vi "Report to logger.vi"(8 "error in (no error)":errorcluster, 10 "Comment":string, 11 "Camera Actor in":refnum<class "Camera Actor.lvclass">) -> (0 "error out":errorcluster, 3 "Camera Actor out":refnum<class "Camera Actor.lvclass">)   [LabVIEW 2020, in "Camera Actor.lvlib" / "Camera Actor.lvclass"]
uses:
  Camera Actor.lvclass
  Camera Actor.lvclass/Camera Actor.ctl
  Logbook/Logbook/Logbook.lvclass
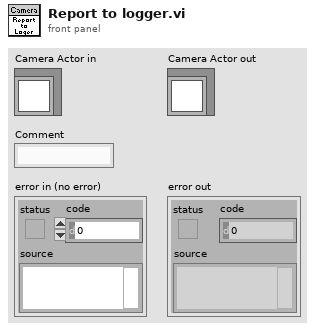
[diagram p1: front panel]
types:
  T1 = typedef "Camera Actor.lvlib/Camera Actor.lvclass/Operation Mode.ctl" = enum16{"Run", "Stop", "Exit", "Error", "Restart"}
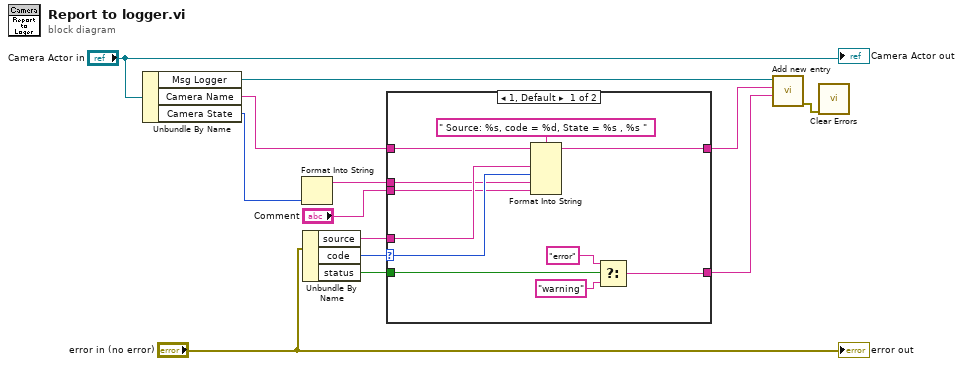
[diagram p0: block diagram]
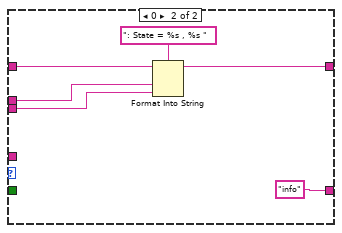
[diagram p2: hidden frame]
diagram:
  n1 = Unbundle By Name("Camera Actor in") -> ("Msg Logger"=w7:refnum<class "Logbook.lvclass">, "Camera Name"=w12:string, "Camera State"=w11:T1)
  n2 = Format Into String(w11) -> (resulting string=w10:string)  [unwired: 3 in, 1 out]
  n3 = Unbundle By Name("error in (no error)") -> ("source"=w3:string, "code"=w2:i32, "status"=w1:bool)
  n4 = case shown="1, Default" w2 {
    selector: w2 -> [w24 _]
    tunnel: w12 -> [w22 w30]
    tunnel: w10 -> [w21 w29]
    tunnel: "Comment" -> [w20 w28]
    tunnel: [w19 w27] -> w5
    tunnel: [w17 "info" ("Severity")] -> w4
    tunnel: w3 -> [w23 _]
    tunnel: w1 -> [w16 _]
    frame 1, Default {
      n5 = Format Into String(format string=" Source: %s, code = %d, State = %s , %s ", initial string=w22, w23, w24, w21, w20) -> (resulting string=w19:string)  [unwired: 1 in, 1 out]
      n6 = Select(t="error" ("Severity"), s=w16, f="warning" ("Severity")) -> (s? t:f=w17:string)
    }
    frame 0 {
      n7 = Format Into String(format string=": State = %s , %s ", initial string=w30, w29, w28) -> (resulting string=w27:string)  [unwired: 1 in, 1 out]
    }
  }
  n8 = call-dynamic "Add new entry.vi"("Severity"=w4, "Text to log"=w5, "Logbook in"=w7) -> ("error out"=w8:errorcluster)  [unwired: 7 in, 1 out]
  n9 = call <vilib>:"Clear Errors.vi"("error in (no error)"=w8) -> ()  [unwired: 5 in, 2 out]
  "error out" <- "error in (no error)"
  "Camera Actor out" <- "Camera Actor in"
